vi "Do.vi"(8 "error in (no error)":errorcluster, 10 "Actor in":refnum<class "Actor.lvclass">, 11 "Write black player Msg":refnum<class "Write black player Msg.lvclass">) -> (0 "error out":errorcluster, 2 "Actor out":refnum<class "Actor.lvclass">)   [LabVIEW 2013, in "GoBang.lvlib" / "Write black player Msg.lvclass"]
doc: "This VI delivers the message to the actor by calling the appropriate method(s) on the actor."
uses:
  Write black player Msg.lvclass
  <vilib>/ActorFramework/Actor/Actor.lvclass
  Client/CS++GoBangClient.lvclass
  Core/Actors/CS++PVMonitor Messages/CS++PVUpdate Msg/CS++PVUpdate Msg.lvclass/CS++PVUpdate Msg.ctl
  Core/Classes/CS++ProcessVariables/ProcessVariable/PV.lvclass/PV.ctl
  Write black player Msg.lvclass/Write black player Msg.ctl
  Core/Actors/CS++PVMonitor Messages/CS++PVUpdate Msg/CS++PVUpdate Msg.lvclass
  Core/Classes/CS++ProcessVariables/ProcessVariable/PV.lvclass
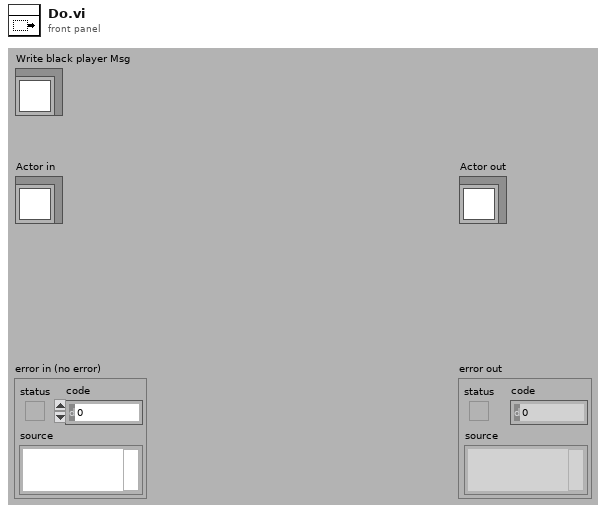
[diagram p1: front panel]
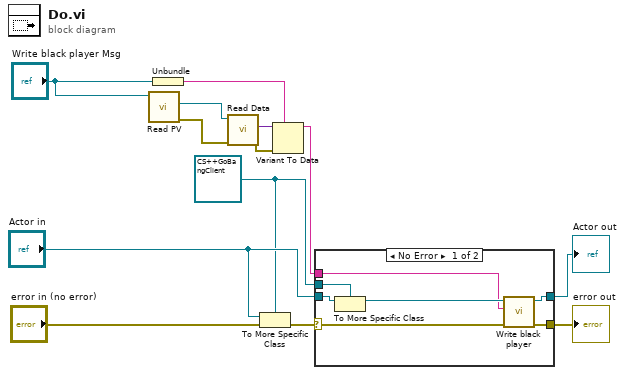
[diagram p0: block diagram]
diagram:
  w8 = refnum<class "CS++GoBangClient.lvclass"> refnum ("Actor in")
  n1 = call "Read PV.vi"("CS++PVUpdate Msg in"="Write black player Msg") -> ("error out"=w4:errorcluster, "PV"=w5:refnum<class "PV.lvclass">)  [unwired: 8 in, 1 out]
  n2 = Unbundle("Write black player Msg") -> (w2:string)
  n3 = call "Read Data.vi"("error in (no error)"=w4, "PV in"=w5) -> ("error out"=w6:errorcluster, "Data"=w7:variant)  [unwired: 7 in, 1 out]
  n4 = To More Specific Class(target class=w8, reference="Actor in", error in="error in (no error)") -> (error out=w12:errorcluster)  [unwired: 1 out]
  n5 = Variant To Data(error in=w6, type=w2, Variant=w7) -> (data=w1:string)  [unwired: 1 out]
  n6 = case shown="No Error" w12 {
    selector: w12 -> [w18 w22]
    tunnel: [w20 w22] -> w11
    tunnel: [w19 w21] -> w10
    tunnel: "Actor in" -> [w17 w21]
    tunnel: w8 -> [w16 _]
    tunnel: w1 -> [w14 _]
    frame No Error {
      n7 = To More Specific Class(target class=w16, reference=w17) -> (specific class reference=w15:refnum<class "CS++GoBangClient.lvclass">)  [unwired: 1 in, 1 out]
      n8 = call-dynamic "Write black player.vi"("error in (no error)"=w18, "BlackPlayer"=w14, "CS++GoBangClient in"=w15) -> ("error out"=w20:errorcluster, "CS++GoBangClient out"=w19:refnum<class "CS++GoBangClient.lvclass">)  [unwired: 7 in]
    }
    frame Error {
      # "If type check fails, pass the original object out again."
    }
  }
  "error out" <- w11
  "Actor out" <- w10
